vi "Unloading.vi"(8 "error In":errorcluster) -> (0 "error out":errorcluster)   [LabVIEW 2017]
uses:
  Controls/UNLOADING_DISPLAY.ctl
  Controls/Unload_Cyc_Data.ctl
  <vilib>/Utility/error.llb/DialogType.ctl
  Controls/QUEUE_STATES.ctl
  Controls/Unload_St.ctl
  <vilib>/Utility/file.llb/Read Delimited Spreadsheet (string).vi
  <vilib>/Instr/_visa.llb/VISA Configure Serial Port (Instr).vi
panel:
  out "EXPECTED SCAN CODE":string
  out "SCANNED CODE STATUS":bool
  out "DOOR OPEN":bool
  out "Cluster":T1
  out "CURRENT PLAN":T2
  out "all rows":string[][](array[string])
  out "logical AND":bool
  out "element":u16
  in  "Close _Door":bool
  out "raw scan code":string
  in  "BYPASS SCN":bool
  in  "String":string
  out "Scanner Comm":bool
  out "Stop scanner":bool
  out "CYCLE STATUS":string
  out "SCAN CODE:":string
  out "Selected Plan structure":string[][](table)
  out "Plan Selected:":string
  out "USER:-":string
  in  "Stop":bool
  out "DATE/TIME":string
  out "Screen Name":string
  # "DOOR NUMBER"
  # "SCANNED CODE"
  # "UNLOAD STATUS"
  # "DOOR NUMBER"
  # "SCANNED CODE"
  # "UNLOAD STATUS"
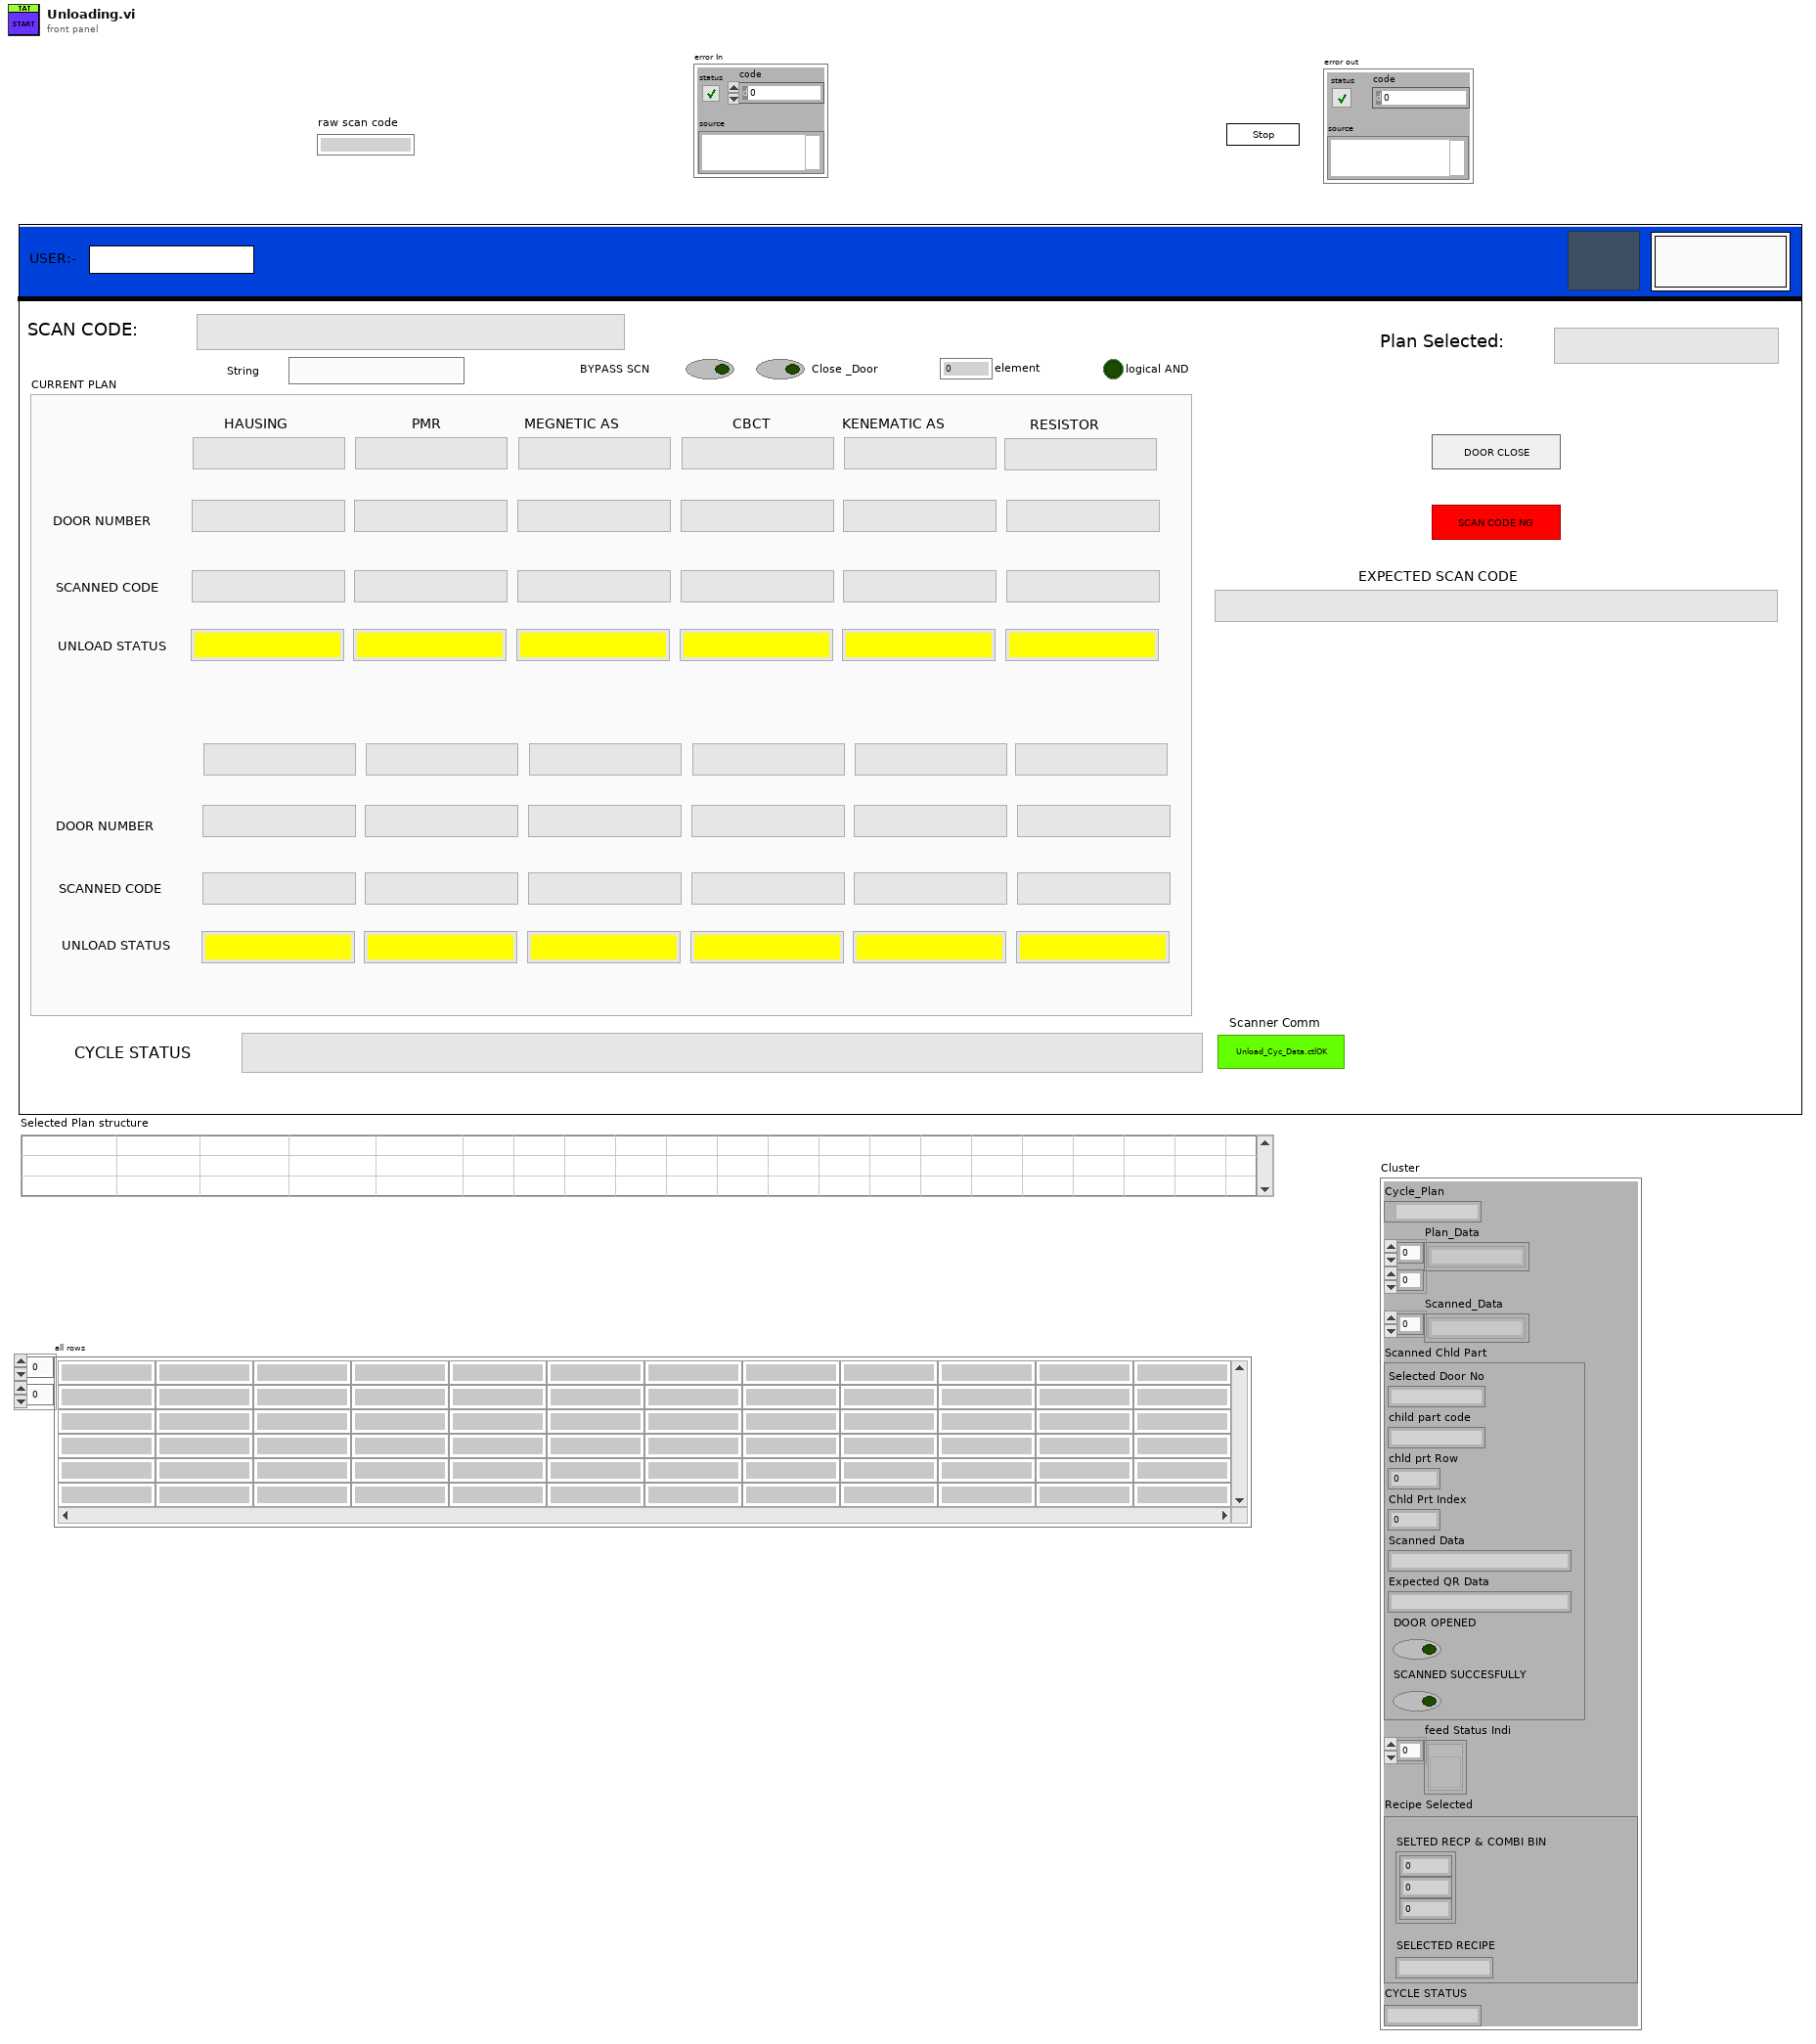
[diagram p1: front panel]
types:
  T1 = typedef "Unload_Cyc_Data.ctl" = cluster{"Cycle_Plan":path, "Plan_Data":string[][], "Scanned_Data":string[], "Scanned Chld Part":cluster{"Selected Door No":string, "child part code":string, "chld prt Row":i32, "Chld Prt Index":i32, "Scanned Data":string, "Expected QR Data":string, "DOOR OPENED":bool, "SCANNED SUCCESFULLY":bool}, "feed Status Indi":refnum<vi>[], "Recipe Selected":cluster{"SELTED RECP & COMBI BIN":cluster{"RECIPE INDEX":i32, "COMBI BIN":i32, "Section row no.":i32}, "SELECTED RECIPE":string}, "CYCLE STATUS":string}
  T2 = typedef "UNLOADING_DISPLAY.ctl" = cluster{"HAUSING":string, "PMR":string, "MEGNETIC AS":string, "CBCT":string, "KENEMATIC AS":string, "RESISTOR":string, "HAUSING DOOR":string, "PMR DOOR":string, "MAGNETIC AS DOOR":string, "CBCT DOOR":string, "KINEMATIC AS DOOR":string, "RESISTOR DOOR":string, "HAUSING SCAN QR":string, "PMR SCAN QR":string, "MAGNETIC SCAN QR":string, "CBCT SCAN QR":string, "KINEMATIC SCAN QR":string, "RESISTOR SCAN QR":string, "HAUSING UNLOAD STATUS":string, "PMR UNLOAD STATUS":string, "MAGNETIC AS UNLOAD STATUS":string, "CBCT UNLOAD STATUS":string, "KINEMATIC AS UNLOAD STATUS":string, "RESISTOR 1 UNLOAD STATUS":string, "HAUSING 2":string, "PMR 2":string, "MEGNETIC AS 2":string, "CBCT 2":string, "KENEMATIC AS 2":string, "RESISTOR 2":string, "HAUSING DOOR 4":string, "PMR DOOR 4":string, "MAGNETIC AS DOOR 4":string, "CBCT DOOR 4":string, "KINEMATIC AS DOOR 4":string, "RESISTOR 1 DOOR 4":string, "HAUSING 2 SCAN QR":string, "PMR 2 SCAN QR":string, "MAGNETIC 2 SCAN QR":string, "CBCT 2 SCAN QR":string, "KINEMATIC 2 SCAN QR":string, "RESISTOR 2 SCAN QR":string, "HAUSING UNLOAD STATUS 2":string, "PMR UNLOAD STATUS 2":string, "MAGNETIC AS UNLOAD STATUS 2":string, "CBCT UNLOAD STATUS 2":string, "KINEMATIC AS UNLOAD STATUS 2":string, "RESISTOR 1 UNLOAD STATUS 2":string}
  T3 = typedef "DialogType.ctl" = u16
  T4 = enum32{"invalid app kind", "Development System", "Run Time System", "Student Edition", "Embedded LabVIEW", "Evaluation", "Custom"}
  T5 = typedef "QUEUE_STATES.ctl" = enum16{"CREATE Q", "EN Q", "DE Q", "CLOSE Q"}
  T6 = cluster{"Printer IP":string, "PLC IP Address":string, "Scanner Com":refnum<visa-resource-name>}
  T7 = typedef "Unload_St.ctl" = enum16{"Int", "Int 2", "Wait", "Cluster_update", "Empty_Bin_Check", "Check_Section_to_Run", "Open_Door", "QR_Scanned", "Close_Door", "Error_Handler", "Stop"}
  T8 = cluster{"RECIPE INDEX":i32, "COMBI BIN":i32, "Section row no.":i32}
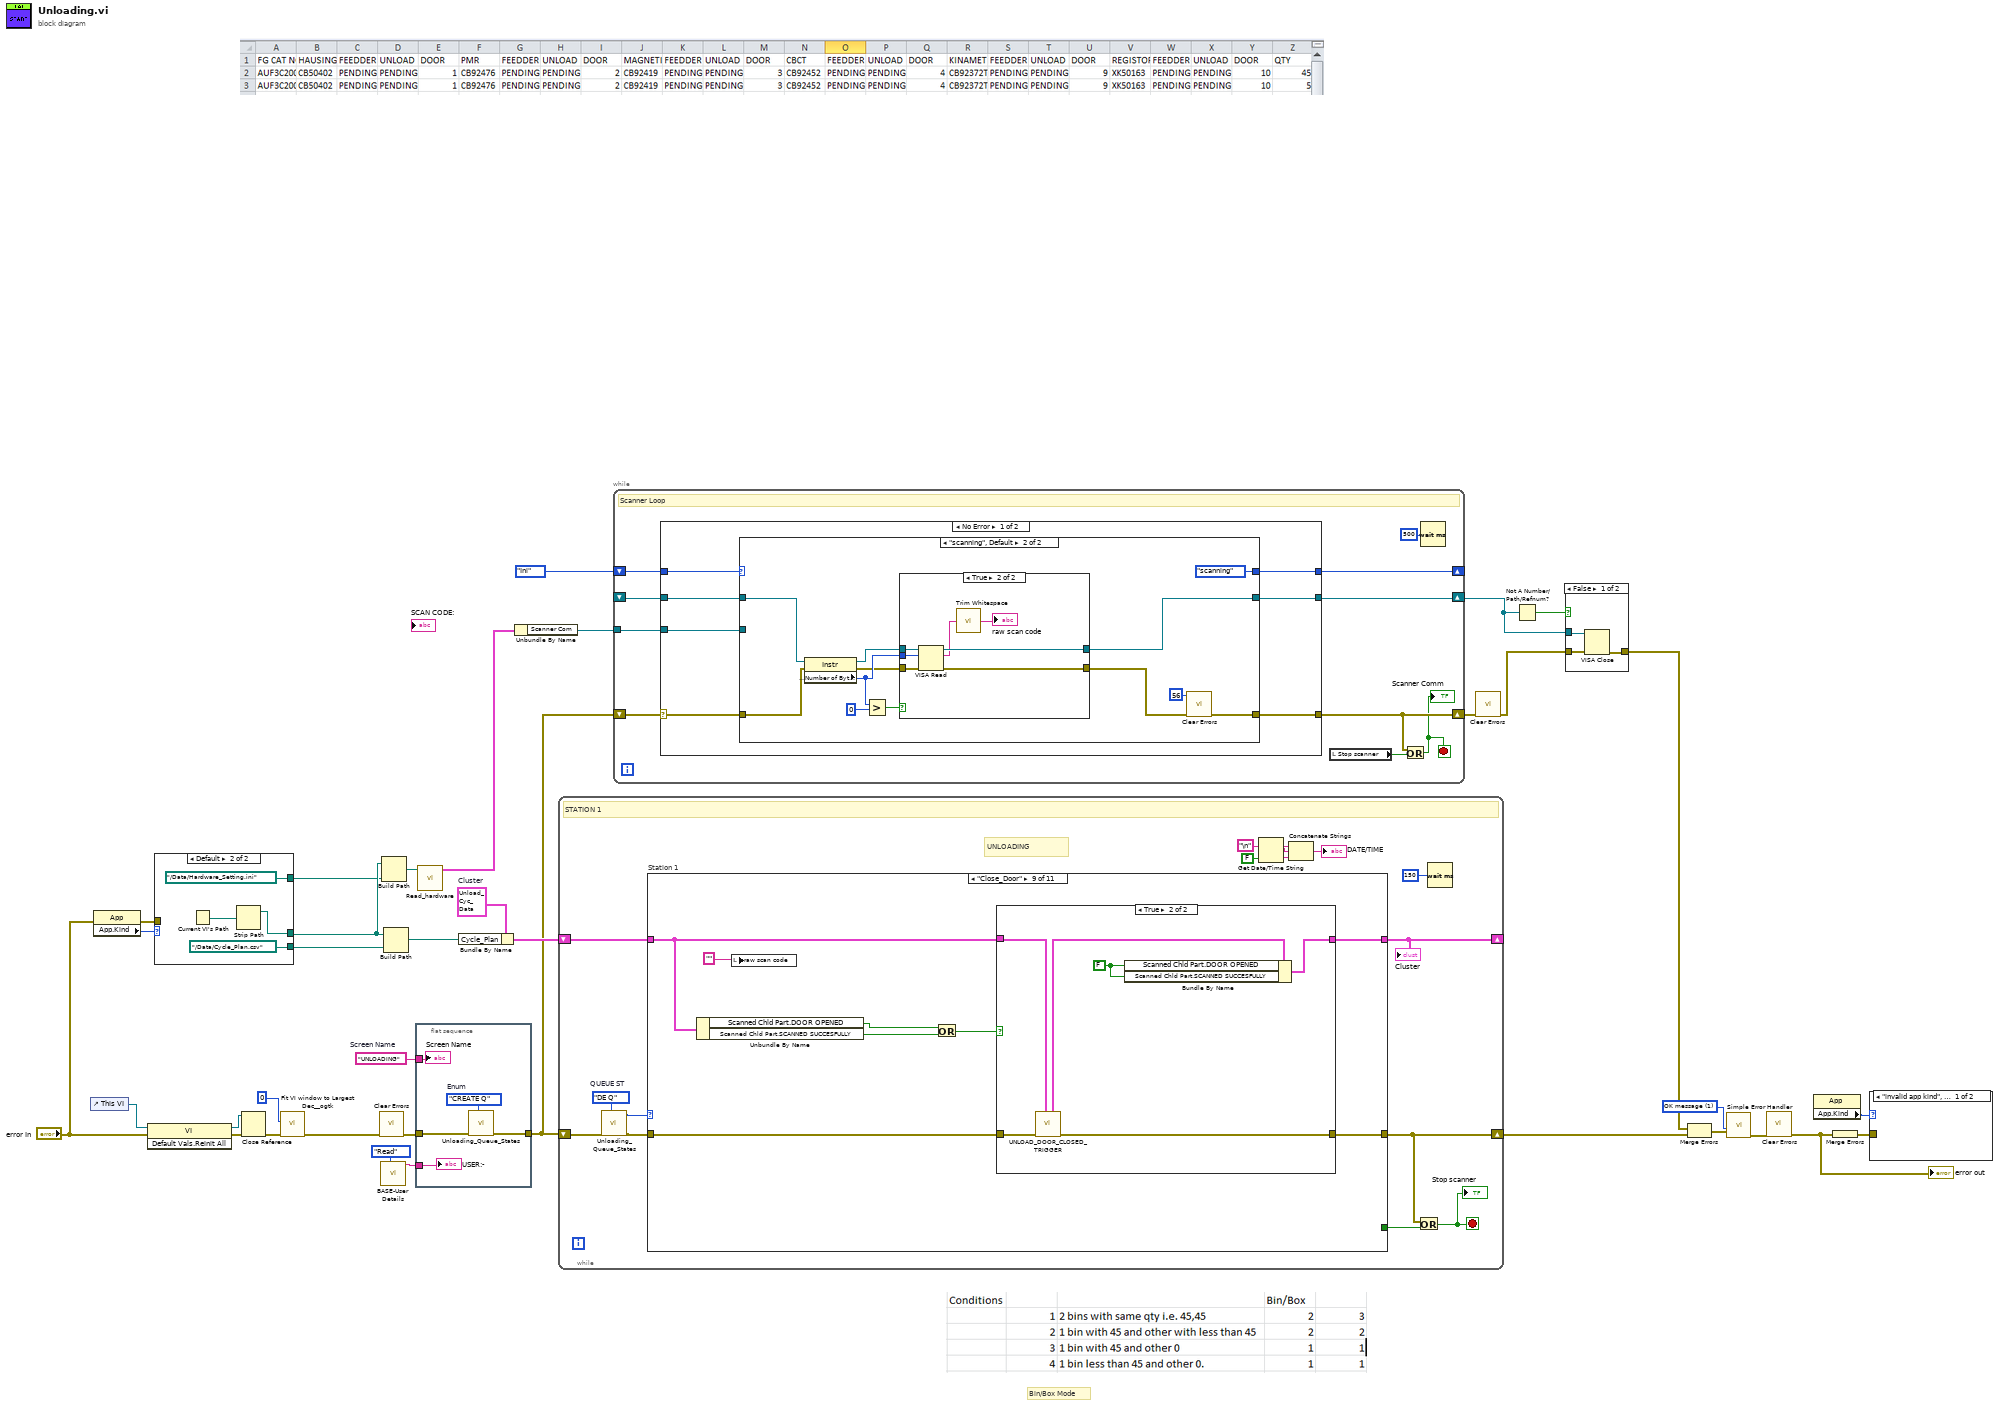
[diagram p0: block diagram]
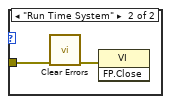
[diagram p2: hidden frame]
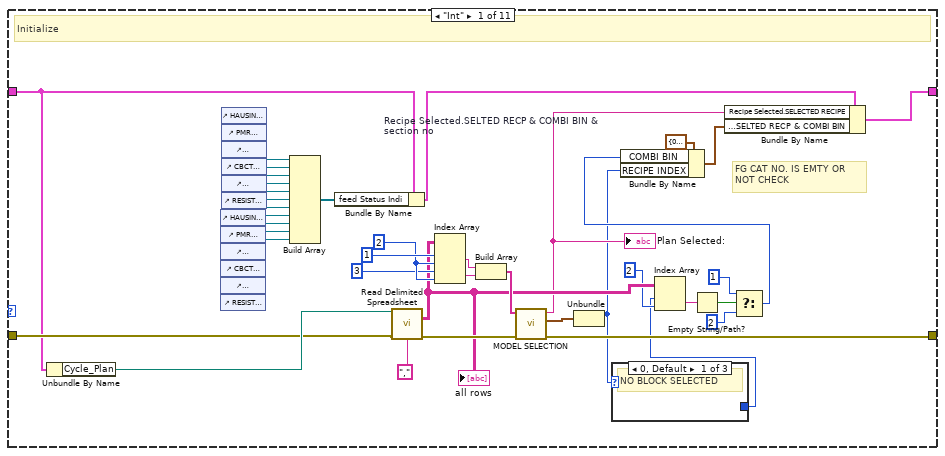
[diagram p3: hidden frame]
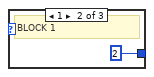
[diagram p4: hidden frame]
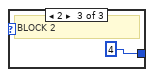
[diagram p5: hidden frame]
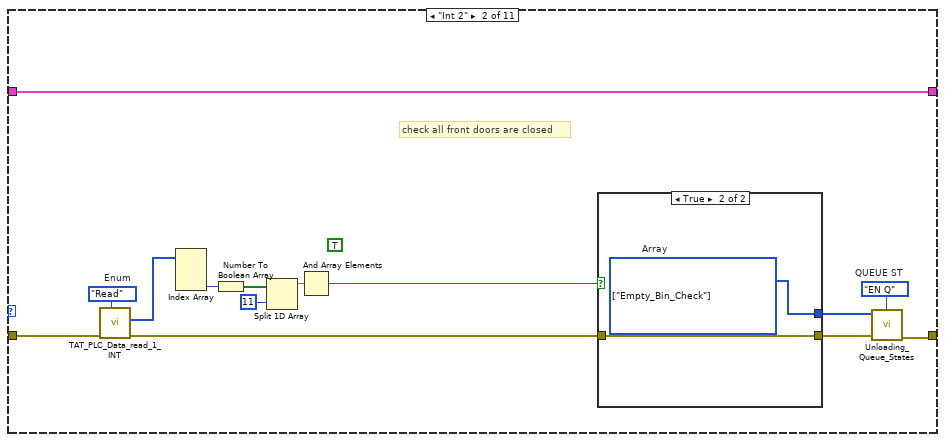
[diagram p6: hidden frame]
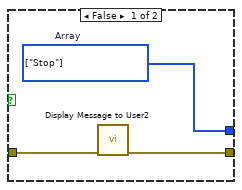
[diagram p7: hidden frame]
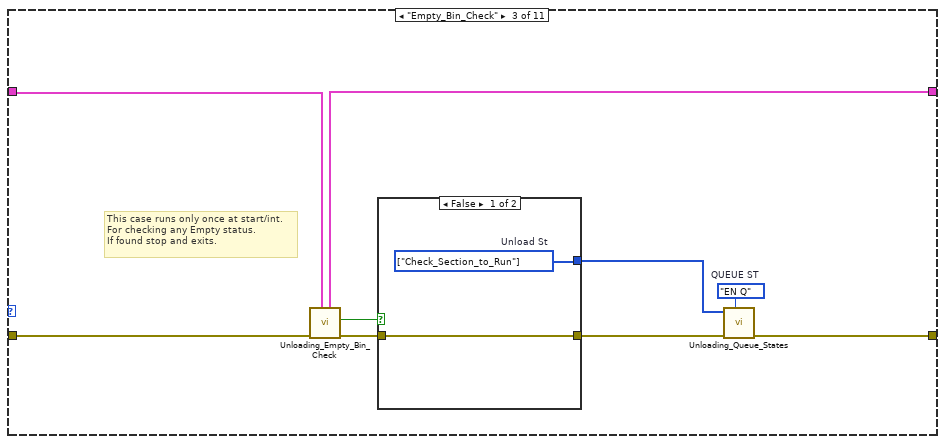
[diagram p8: hidden frame]
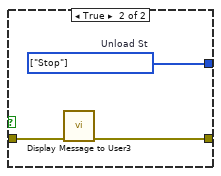
[diagram p9: hidden frame]
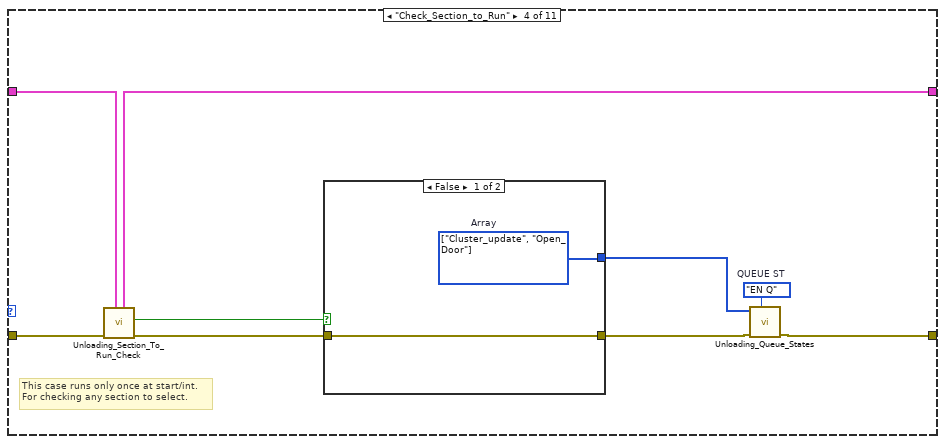
[diagram p10: hidden frame]
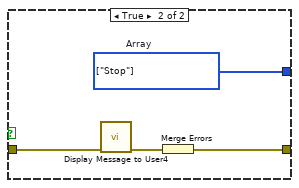
[diagram p11: hidden frame]
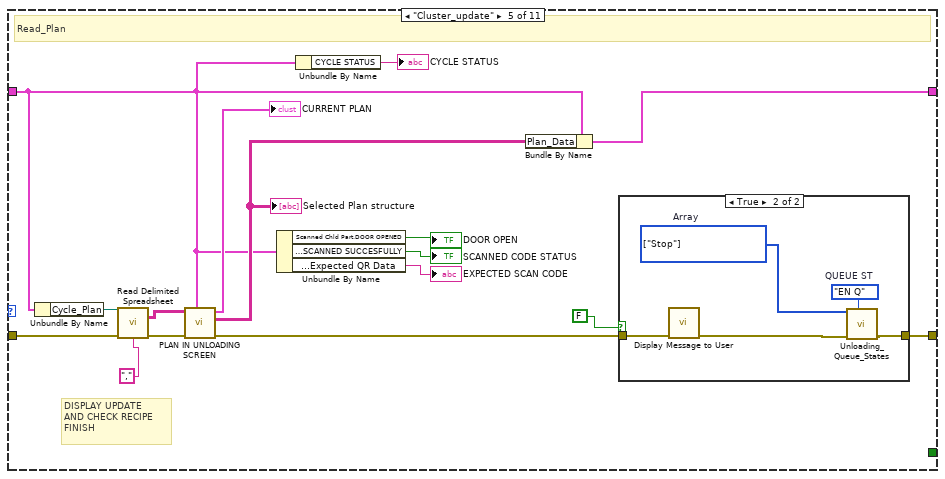
[diagram p12: hidden frame]
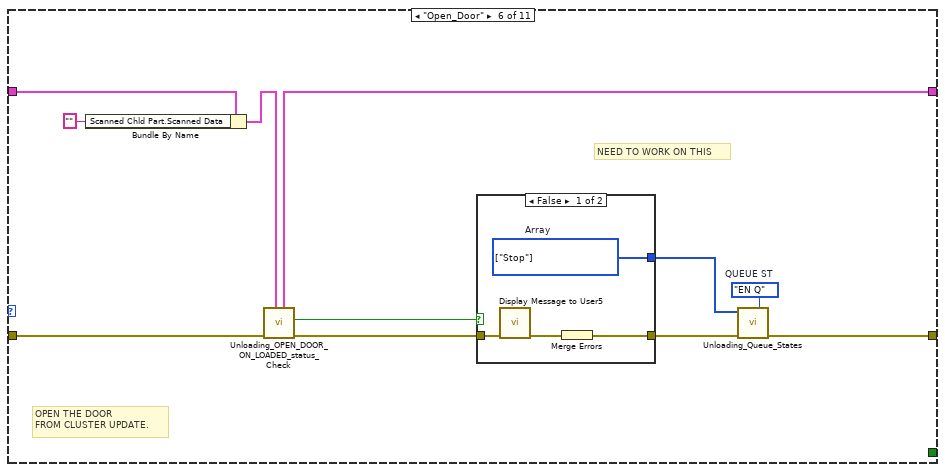
[diagram p14: hidden frame]
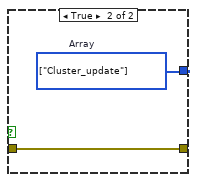
[diagram p15: hidden frame]
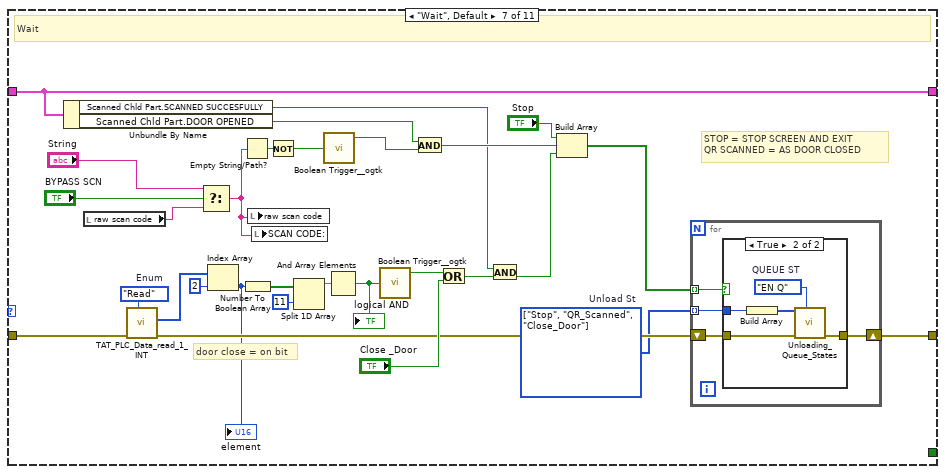
[diagram p16: hidden frame]
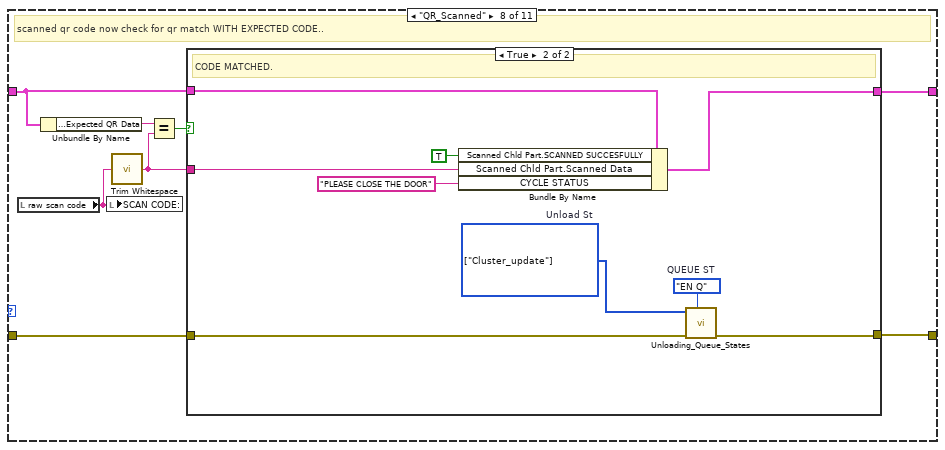
[diagram p18: hidden frame]
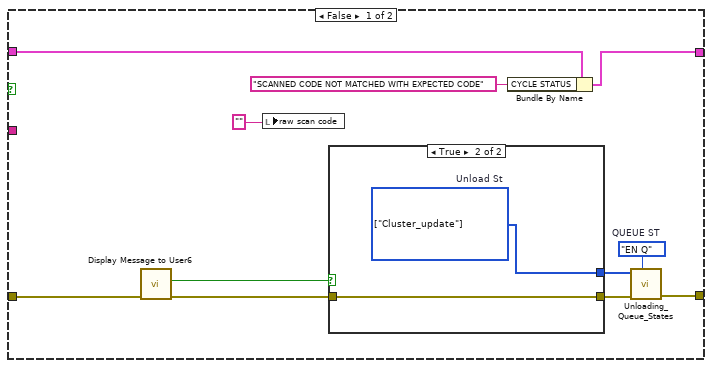
[diagram p19: hidden frame]
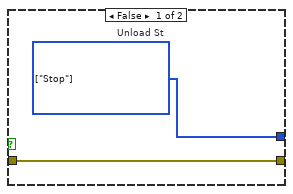
[diagram p20: hidden frame]
diagram:
  w1 = T1 {"Cycle_Plan"=path "", "Plan_Data"=[], "Scanned_Data"=[], "Scanned Chld Part"={"Selected Door No"="", "child part code"="", "chld prt Row"=0, "Chld Prt Index"=0, "Scanned Data"="", "Expected QR Data"="", "DOOR OPENED"=FALSE, "SCANNED SUCCESFULLY"=FALSE}, "feed Status Indi"=[], "Recipe Selected"={"SELTED RECP & COMBI BIN"={"RECIPE INDEX"=0, "COMBI BIN"=0, "Section row no."=0}, "SELECTED RECIPE"=""}, "CYCLE STATUS"=""}  # Cluster
  w18 = "UNLOADING"  # Screen Name
  w29 = T3 1 items=["no dialog", "OK message", "continue or stop message", "OK message + warnings", "continue/stop + warnings"] ("type of dialog (OK msg:1)")
  # "Bin/Box Mode"
  n1 = control-ref of="This VI"() -> (w36:refnum<vi>)
  n2 = property class="App"(error in="error In") -> (error out=w25:errorcluster, "App.Kind"=w27:T4)  [unwired: 1 in, 1 out]
  n3 = invoke class="VI" method="Default Vals.Reinit All"(reference=w36, error in="error In") -> (reference out=w34:refnum<vi>, error out=w35:errorcluster)  [unwired: 1 in, 1 out]
  n4 = case shown="Default" w27 {
    tunnel: [path "Data/Cycle_Plan.csv" ("path") path "../Data/Cycle_Plan.csv" ("path")] -> w26
    tunnel: [w37 w41] -> w7
    tunnel: w25 -> [_ _]
    tunnel: [path "Data/Hardware_Setting.ini" ("path") path "../Data/Hardware_Setting.ini" ("path")] -> w6
    frame "Run Time System" {
      n5 = call <vilib>:"Application Directory.vi"() -> ("Application Directory"=w37:path)
    }
    frame Default {
      n6 = Current VI's Path() -> (path=w42:path)
      n7 = Strip Path(path=w42) -> (stripped path=w41:path)  [unwired: 1 out]
    }
  }
  n8 = Close Reference(reference=w34, error in (no error)=w35) -> (error out=w33:errorcluster)
  n9 = call <userlib>:"Fit VI window to Largest Dec__ogtk.vi"("error in (no error)"=w33, "border spacing (2 px)"=0) -> ("error out"=w23:errorcluster)  [unwired: 4 in, 1 out]
  n10 = call <vilib>:"Clear Errors.vi"("error in (no error)"=w23) -> ("error out"=w11:errorcluster)  [unwired: 5 in, 1 out]
  n11 = call "BASE-User Details.vi"("Enum"=enum16{"Read", "Write"}."Read") -> ("User Name Out"=w30:string)  [unwired: 9 in, 1 out]
  n12 = Build Path(base path=w7, name or relative path=w6) -> (appended path=w5:path)
  n13 = Build Path(base path=w7, name or relative path=w26) -> (appended path=w20:path)
  n14 = flat-sequence {
    tunnel: [w45] -> w12
    tunnel: w11 -> [w46]
    tunnel: w30 -> [w48]
    tunnel: w18 -> [w47]
    frame #0 {
      w44 = QUEUE_STATES."CREATE Q"  # Enum
      n15 = call "Unloading_Queue_States.vi"("QUEUE ST"=w44, "error in"=w46) -> ("error OUT"=w45:errorcluster)  [unwired: 8 in, 1 out]
      "USER:-" <- w48
      "Screen Name" <- w47
    }
  }
  n16 = call "Read_hardware.vi"("configuration file path"=w5) -> ("data"=w9:T6)  [unwired: 10 in]
  n17 = Bundle By Name(cluster=w1, "Cycle_Plan"=w20) -> (w19:T1)
  n18 = Unbundle By Name(w9) -> ("Scanner Com"=w8:refnum<visa-resource-name>)
  n19 = while {
    shift-right: [w55] -> _
    shift-left: w19 -> [w56]
    shift-right: [w53] -> w10
    shift-left: w12 -> [w52]
    stop <- w54 stop-if-true
    w49 = QUEUE_STATES."DE Q"  # QUEUE ST
    # "UNLOADING"
    # "STATION 1"
    n20 = call "Unloading_Queue_States.vi"("QUEUE ST"=w49, "error in"=w52) -> ("error OUT"=w51:errorcluster, "Unload ST"=w50:T7)  [unwired: 8 in]
    n21 = case "Station 1" shown="\"Close_Door\"" w50 {
      tunnel: [_ _ _ _ _ _ _ _ _ _ TRUE] -> w57
      tunnel: [w80 w108 w128 w145 w158 w176 w218 w238 w269 w284 w288] -> w53
      tunnel: w51 -> [w98 w112 w132 w143 w167 w183 w209 w236 w270 w285 w289]
      tunnel: w56 -> [w89 w118 w131 w141 w156 w182 w196 w235 w268 w283 w290]
      tunnel: [w90 w118 w130 w140 w159 w181 w196 w237 w267 w283 w290] -> w55
      frame "Int" {
        w68 = T8 {"RECIPE INDEX"=0, "COMBI BIN"=0, "Section row no."=0}  # Recipe Selected.SELTED RECP & COMBI BIN & section no
        w95 = 2
        # "FG CAT NO. IS EMTY OR \nNOT CHECK"
        # "Initialize"
        n22 = Unbundle By Name(w89) -> ("Cycle_Plan"=w101:path)
        n23 = control-ref of="HAUSING UNLOAD STATUS 2"() -> (w73:refnum<vi>)
        n24 = control-ref of="PMR UNLOAD STATUS 2"() -> (w72:refnum<vi>)
        n25 = control-ref of="MAGNETIC AS UNLOAD STATUS 2"() -> (w71:refnum<vi>)
        n26 = control-ref of="CBCT UNLOAD STATUS 2"() -> (w70:refnum<vi>)
        n27 = control-ref of="KINEMATIC AS UNLOAD STATUS 2"() -> (w69:refnum<vi>)
        n28 = control-ref of="RESISTOR 1 UNLOAD STATUS 2"() -> ()  [unwired: 1 out]
        n29 = control-ref of="HAUSING UNLOAD STATUS"() -> (w79:refnum<vi>)
        n30 = control-ref of="PMR UNLOAD STATUS"() -> (w78:refnum<vi>)
        n31 = control-ref of="MAGNETIC AS UNLOAD STATUS"() -> (w77:refnum<vi>)
        n32 = control-ref of="CBCT UNLOAD STATUS"() -> (w76:refnum<vi>)
        n33 = control-ref of="KINEMATIC AS UNLOAD STATUS"() -> (w75:refnum<vi>)
        n34 = control-ref of="RESISTOR 1 UNLOAD STATUS"() -> (w74:refnum<vi>)
        n35 = Build Array(w79, w78, w77, w76, w75, w74, w73, w72, w71, w70, w69) -> (w102:refnum<vi>[])
        n36 = Bundle By Name(cluster=w89, "feed Status Indi"=w102) -> (w91:T1)
        n37 = call-poly <vilib>:"Read Delimited Spreadsheet.vi"("file path (dialog if empty)"=w101, "error in (no error)"=w98, "delimiter (\\t)"=",") -> ("all rows"=w88:string[][], "error out"=w97:errorcluster)  [unwired: 7 in, 4 out]
        "all rows" <- w88
        n38 = Index Array(array=w88, index (row) #1=1, index (col) #1=w95, index (row) #2=3, index (col) #2=w95) -> (element #1=w93:string, element #2=w92:string)
        n39 = Build Array(w93, w92) -> (w100:string[])
        n40 = call "MODEL SELECTION.vi"("error in (no error)"=w97, "Plan List"=w100) -> ("error out 2"=w80:errorcluster, "SELECTED RECIPE\nand COMBI OF BIN- INDEX"=w82:cluster{"RECIPE INDEX":i32, "COMBI BIN":i32}, "Plan Selected"=w81:string)  [unwired: 7 in]
        "Plan Selected:" <- w81
        n41 = Unbundle(w82) -> ("RECIPE INDEX"=w64:i32)  [unwired: 1 out]
        n42 = case shown="0, Default" w64 {
          tunnel: [_ 2 4] -> w65
          frame 0, Default {
            # "NO BLOCK SELECTED"
          }
          frame 1 {
            # "BLOCK 1"
          }
          frame 2 {
            # "BLOCK 2"
          }
        }
        n43 = Index Array(array=w88, index (row)=w65, index (col)=2) -> (element=w86:string)
        n44 = Empty String/Path?(string/path=w86) -> (empty?=w85:bool)
        n45 = Select(t=1, s=w85, f=2) -> (s? t:f=w66:i32)
        n46 = Bundle By Name(cluster=w68, "COMBI BIN"=w66, "RECIPE INDEX"=w64) -> (w67:T8)
        n47 = Bundle By Name(cluster=w91, "Recipe Selected.SELECTED RECIPE"=w81, "Recipe Selected.SELTED RECP & COMBI BIN"=w67) -> (w90:T1)
      }
      frame "Int 2" {
        (unwired) TRUE
        w110 = QUEUE_STATES."EN Q"  # QUEUE ST
        w117 = enum16{"Read", "Write"}."Read"  # Enum
        # "check all front doors are closed"
        n48 = call "TAT_PLC_Data_read_1_INT.vi"("Enum"=w117, "error in (no error)"=w112) -> ("error out"=w111:errorcluster, "Array 2"=w116:u16[])  [unwired: 8 in]
        n49 = Index Array(array=w116) -> (element #3=w105:u16)  [unwired: 3 in, 2 out]
        n50 = Number To Boolean Array(number=w105) -> (Boolean array=w115:bool[])
        n51 = Split 1D Array(array=w115, index=11) -> (first subarray=w113:bool[])  [unwired: 1 out]
        n52 = And Array Elements(Boolean array=w113) -> (logical AND=w106:bool)
        n53 = case shown="True" w106 {
          tunnel: w111 -> [w121 w123]
          tunnel: [w120 w123] -> w107
          tunnel: [w119 w122] -> w109
          frame False {
            w119 = T7[] [enum."Stop"] items=["Int", "Int 2", "Wait", "Cluster_update", "Empty_Bin_Check", "Check_Section_to_Run", "Open_Door", "QR_Scanned", "Close_Door", "Error_Handler", "Stop"]  # Array
            n54 = call "Display Message to User2"("error in (no error)"=w121) -> ("error out"=w120:errorcluster)  [unwired: 9 in, 1 out]
          }
          frame True {
            w122 = T7[] [enum."Empty_Bin_Check"] items=["Int", "Int 2", "Wait", "Cluster_update", "Empty_Bin_Check", "Check_Section_to_Run", "Open_Door", "QR_Scanned", "Close_Door", "Error_Handler", "Stop"]  # Array
          }
        }
        n55 = call "Unloading_Queue_States.vi"("QUEUE ST"=w110, "error in"=w107, "Unload St"=w109) -> ("error OUT"=w108:errorcluster)  [unwired: 7 in, 1 out]
      }
      frame "Empty_Bin_Check" {
        w127 = QUEUE_STATES."EN Q"  # QUEUE ST
        # "This case runs only once at start/int.\nFor checking any Empty status.\nIf found stop and exits."
        n56 = call "Unloading_Empty_Bin_Check.vi"("Cluster DATA IN"=w131, "error in (no error)"=w132) -> ("error out"=w129:errorcluster, "EMPTY FOUND ?"=w124:bool, "Cluster DATA OUT"=w130:T1)  [unwired: 7 in]
        n57 = case shown="False" w124 {
          tunnel: w129 -> [w134 w137]
          tunnel: [w133 w136] -> w126
          tunnel: [w134 w135] -> w125
          frame False {
            w133 = T7[] [enum."Check_Section_to_Run"] items=["Int", "Int 2", "Wait", "Cluster_update", "Empty_Bin_Check", "Check_Section_to_Run", "Open_Door", "QR_Scanned", "Close_Door", "Error_Handler", "Stop"]  # Unload St
          }
          frame True {
            w136 = T7[] [enum."Stop"] items=["Int", "Int 2", "Wait", "Cluster_update", "Empty_Bin_Check", "Check_Section_to_Run", "Open_Door", "QR_Scanned", "Close_Door", "Error_Handler", "Stop"]  # Unload St
            n58 = call "Display Message to User3"("error in (no error)"=w137) -> ("error out"=w135:errorcluster)  [unwired: 9 in, 1 out]
          }
        }
        n59 = call "Unloading_Queue_States.vi"("QUEUE ST"=w127, "error in"=w125, "Unload St"=w126) -> ("error OUT"=w128:errorcluster)  [unwired: 7 in, 1 out]
      }
      frame "Check_Section_to_Run" {
        w146 = QUEUE_STATES."EN Q"  # QUEUE ST
        # "This case runs only once at start/int.\nFor checking any section to select."
        n60 = call "Unloading_Section_To_Run_Check.vi"("Cluster DATA IN"=w141, "error in (no error)"=w143) -> ("error out"=w142:errorcluster, "FULLY UNLOADED FOUND ?"=w138:bool, "Cluster DATA OUT"=w140:T1)  [unwired: 7 in]
        n61 = case shown="False" w138 {
          tunnel: [w148 w152] -> w144
          tunnel: w142 -> [w147 w150]
          tunnel: [w147 w151] -> w139
          frame False {
            w148 = T7[] [enum."Cluster_update", enum."Open_Door"] items=["Int", "Int 2", "Wait", "Cluster_update", "Empty_Bin_Check", "Check_Section_to_Run", "Open_Door", "QR_Scanned", "Close_Door", "Error_Handler", "Stop"]  # Array
          }
          frame True {
            w152 = T7[] [enum."Stop"] items=["Int", "Int 2", "Wait", "Cluster_update", "Empty_Bin_Check", "Check_Section_to_Run", "Open_Door", "QR_Scanned", "Close_Door", "Error_Handler", "Stop"]  # Array
            n62 = call "Display Message to User4"("error in (no error)"=w150) -> ("error out"=w149:errorcluster)  [unwired: 9 in, 1 out]
            n63 = Merge Errors(w149) -> (w151:errorcluster)
          }
        }
        n64 = call "Unloading_Queue_States.vi"("QUEUE ST"=w146, "error in"=w139, "Unload St"=w144) -> ("error OUT"=w145:errorcluster)  [unwired: 7 in, 1 out]
      }
      frame "Cluster_update" {
        # "DISPLAY UPDATE\nAND CHECK RECIPE\nFINISH"
        # "Read_Plan"
        n65 = Unbundle By Name(w156) -> ("Cycle_Plan"=w166:path)
        n66 = call-poly <vilib>:"Read Delimited Spreadsheet.vi"("file path (dialog if empty)"=w166, "error in (no error)"=w167, "delimiter (\\t)"=",") -> ("all rows"=w162:string[][], "error out"=w164:errorcluster)  [unwired: 7 in, 4 out]
        n67 = call "PLAN IN UNLOADING SCREEN.vi"("LOOP DATA IN"=w156, "error IN"=w164, "PLAN In"=w162) -> ("error out"=w163:errorcluster, "PLAN Out"=w160:string[][], "CURRENT PLAN"=→"CURRENT PLAN":T2)  [unwired: 4 in, 1 out]
        "Selected Plan structure" <- w160
        n68 = Unbundle By Name(w156) -> ("Scanned Chld Part.DOOR OPENED"=→"DOOR OPEN":bool, "Scanned Chld Part.SCANNED SUCCESFULLY"=→"SCANNED CODE STATUS":bool, "Scanned Chld Part.Expected QR Data"=→"EXPECTED SCAN CODE":string)
        n69 = Unbundle By Name(w156) -> ("CYCLE STATUS"=→"CYCLE STATUS":string)
        n70 = Bundle By Name(cluster=w156, "Plan_Data"=w160) -> (w159:T1)
        n71 = case shown="True" FALSE {
          tunnel: w163 -> [w169 w174]
          tunnel: [w169 w171] -> w158
          frame False {
          }
          frame True {
            w170 = T7[] [enum."Stop"] items=["Int", "Int 2", "Wait", "Cluster_update", "Empty_Bin_Check", "Check_Section_to_Run", "Open_Door", "QR_Scanned", "Close_Door", "Error_Handler", "Stop"]  # Array
            w173 = QUEUE_STATES."EN Q"  # QUEUE ST
            n72 = call "Display Message to User"("error in (no error)"=w174) -> ("error out"=w172:errorcluster)  [unwired: 9 in, 1 out]
            n73 = call "Unloading_Queue_States.vi"("QUEUE ST"=w173, "error in"=w172, "Unload St"=w170) -> ("error OUT"=w171:errorcluster)  [unwired: 7 in, 1 out]
          }
        }
      }
      frame "Open_Door" {
        w178 = QUEUE_STATES."EN Q"  # QUEUE ST
        # "NEED TO WORK ON THIS"
        # "OPEN THE DOOR\nFROM CLUSTER UPDATE."
        n74 = Bundle By Name(cluster=w182, "Scanned Chld Part.Scanned Data"="") -> (w185:T1)
        n75 = call "Unloading_OPEN_DOOR_ON_LOADED_status_Check.vi"("CYCLE DATA IN"=w185, "error in"=w183) -> ("error out"=w177:errorcluster, "search valid ?"=w175:bool, "CYCLE DATA OUT"=w181:T1)  [unwired: 7 in]
        n76 = case shown="False" w175 {
          tunnel: [w189 w191] -> w180
          tunnel: w177 -> [w187 w190]
          tunnel: [w188 w190] -> w179
          frame False {
            w189 = T7[] [enum."Stop"] items=["Int", "Int 2", "Wait", "Cluster_update", "Empty_Bin_Check", "Check_Section_to_Run", "Open_Door", "QR_Scanned", "Close_Door", "Error_Handler", "Stop"]  # Array
            n77 = call "Display Message to User5"("error in (no error)"=w187) -> ("error out"=w186:errorcluster)  [unwired: 9 in, 1 out]
            n78 = Merge Errors(w186) -> (w188:errorcluster)
          }
          frame True {
            w191 = T7[] [enum."Cluster_update"] items=["Int", "Int 2", "Wait", "Cluster_update", "Empty_Bin_Check", "Check_Section_to_Run", "Open_Door", "QR_Scanned", "Close_Door", "Error_Handler", "Stop"]  # Array
          }
        }
        n79 = call "Unloading_Queue_States.vi"("QUEUE ST"=w178, "error in"=w179, "Unload St"=w180) -> ("error OUT"=w176:errorcluster)  [unwired: 7 in, 1 out]
      }
      frame "Wait", Default {
        w192 = T7[] [enum."Stop", enum."QR_Scanned", enum."Close_Door"] items=["Int", "Int 2", "Wait", "Cluster_update", "Empty_Bin_Check", "Check_Section_to_Run", "Open_Door", "QR_Scanned", "Close_Door", "Error_Handler", "Stop"]  # Unload St
        w207 = enum16{"Read", "Write"}."Read"  # Enum
        # "STOP = STOP SCREEN AND EXIT\nQR SCANNED = AS DOOR CLOSED"
        # "door close = on bit"
        # "Wait"
        n80 = Unbundle By Name(w196) -> ("Scanned Chld Part.SCANNED SUCCESFULLY"=w193:bool, "Scanned Chld Part.DOOR OPENED"=w195:bool)
        n81 = local read "raw scan code"() -> (w214:string)
        n82 = call "TAT_PLC_Data_read_1_INT.vi"("Enum"=w207, "error in (no error)"=w209) -> ("error out"=w208:errorcluster, "Array 2"=w206:u16[])  [unwired: 8 in]
        n83 = Select(t="String", s="BYPASS SCN", f=w214) -> (s? t:f=w211:string)
        n84 = Index Array(array=w206, index=2) -> (element=w203:u16)
        "element" <- w203
        n85 = Empty String/Path?(string/path=w211) -> (empty?=w217:bool)
        n86 = Number To Boolean Array(number=w203) -> (Boolean array=w202:bool[])
        n87 = local write "raw scan code"(w211) -> ()
        n88 = local write "SCAN CODE:"(w211) -> ()
        n89 = Not(x=w217) -> (.not. x?=w210:bool)
        n90 = Split 1D Array(array=w202, index=11) -> (first subarray=w200:bool[])  [unwired: 1 out]
        n91 = call <userlib>:"Boolean Trigger__ogtk.vi"("Boolean Input"=w210) -> ("Rising Edge"=w205:bool)  [unwired: 1 in, 1 out]
        n92 = And Array Elements(Boolean array=w200) -> (logical AND=w197:bool)
        "logical AND" <- w197
        n93 = call <userlib>:"Boolean Trigger__ogtk.vi"("Boolean Input"=w197) -> ("Rising Edge"=w204:bool)  [unwired: 1 in, 1 out]
        n94 = And(x=w195, y=w205) -> (x .and. y?=w198:bool)
        n95 = Or(x=w204, y="Close _Door") -> (x .or. y?=w212:bool)
        n96 = And(x=w193, y=w212) -> (x .and. y?=w194:bool)
        n97 = Build Array("Stop", w198, w194) -> (w215:bool[])
        n98 = for {
          shift-right: [w223] -> w218
          shift-left: w208 -> [w224]
          tunnel: w215 -> [w222] mode=indexing
          tunnel: w192 -> [w221] mode=indexing
          n99 = case shown="True" w222 {
            tunnel: w224 -> [w225 w228]
            tunnel: [w225 w229] -> w223
            tunnel: w221 -> [_ w230]
            frame False {
            }
            frame True {
              w227 = QUEUE_STATES."EN Q"  # QUEUE ST
              n100 = Build Array(w230) -> (w226:T7[])
              n101 = call "Unloading_Queue_States.vi"("QUEUE ST"=w227, "error in"=w228, "Unload St"=w226) -> ("error OUT"=w229:errorcluster)  [unwired: 7 in, 1 out]
            }
          }
        }
      }
      frame "QR_Scanned" {
        # "scanned qr code now check for qr match WITH EXPECTED CODE.."
        n102 = local read "raw scan code"() -> (w233:string)
        n103 = Unbundle By Name(w235) -> ("Scanned Chld Part.Expected QR Data"=w234:string)
        n104 = local write "SCAN CODE:"(w233) -> ()
        n105 = call <vilib>:"Trim Whitespace.vi"("string"=w233) -> ("trimmed string"=w231:string)  [unwired: 1 in]
        n106 = Equal?(x=w234, y=w231) -> (x = y?=w232:bool)
        n107 = case shown="True" w232 {
          tunnel: [w241 w255] -> w238
          tunnel: [w248 w261] -> w237
          tunnel: w236 -> [w246 w256]
          tunnel: w235 -> [w249 w262]
          tunnel: w231 -> [_ w259]
          frame False {
            w242 = QUEUE_STATES."EN Q"  # QUEUE ST
            n108 = call "Display Message to User6"("error in (no error)"=w246) -> ("error out"=w245:errorcluster, "RETRY"=w244:bool)  [unwired: 9 in]
            n109 = local write "raw scan code"("") -> ()
            n110 = case shown="True" w244 {
              tunnel: w245 -> [w251 w253]
              tunnel: [w251 w253] -> w240
              tunnel: [w250 w252] -> w239
              frame False {
                w250 = T7[] [enum."Stop"] items=["Int", "Int 2", "Wait", "Cluster_update", "Empty_Bin_Check", "Check_Section_to_Run", "Open_Door", "QR_Scanned", "Close_Door", "Error_Handler", "Stop"]  # Unload St
              }
              frame True {
                w252 = T7[] [enum."Cluster_update"] items=["Int", "Int 2", "Wait", "Cluster_update", "Empty_Bin_Check", "Check_Section_to_Run", "Open_Door", "QR_Scanned", "Close_Door", "Error_Handler", "Stop"]  # Unload St
              }
            }
            n111 = Bundle By Name(cluster=w249, "CYCLE STATUS"="SCANNED CODE NOT MATCHED WITH EXPECTED CODE") -> (w248:T1)
            n112 = call "Unloading_Queue_States.vi"("QUEUE ST"=w242, "error in"=w240, "Unload St"=w239) -> ("error OUT"=w241:errorcluster)  [unwired: 7 in, 1 out]
          }
          frame True {
            w257 = QUEUE_STATES."EN Q"  # QUEUE ST
            w254 = T7[] [enum."Cluster_update"] items=["Int", "Int 2", "Wait", "Cluster_update", "Empty_Bin_Check", "Check_Section_to_Run", "Open_Door", "QR_Scanned", "Close_Door", "Error_Handler", "Stop"]  # Unload St
            # "CODE MATCHED."
            n113 = Bundle By Name(cluster=w262, "Scanned Chld Part.SCANNED SUCCESFULLY"=TRUE, "Scanned Chld Part.Scanned Data"=w259, "CYCLE STATUS"="PLEASE CLOSE THE DOOR") -> (w261:T1)
            n114 = call "Unloading_Queue_States.vi"("QUEUE ST"=w257, "error in"=w256, "Unload St"=w254) -> ("error OUT"=w255:errorcluster)  [unwired: 7 in, 1 out]
          }
        }
      }
      frame "Close_Door" {
        n115 = Unbundle By Name(w268) -> ("Scanned Chld Part.DOOR OPENED"=w264:bool, "Scanned Chld Part.SCANNED SUCCESFULLY"=w266:bool)
        n116 = local write "raw scan code"("") -> ()
        n117 = Or(x=w264, y=w266) -> (x .or. y?=w265:bool)
        n118 = case shown="True" w265 {
          tunnel: w270 -> [w276 w282]
          tunnel: [w271 w281] -> w269
          tunnel: w268 -> [w275 w280]
          tunnel: [w275 w278] -> w267
          frame False {
            w273 = T7[] [enum."Stop"] items=["Int", "Int 2", "Wait", "Cluster_update", "Empty_Bin_Check", "Check_Section_to_Run", "Open_Door", "QR_Scanned", "Close_Door", "Error_Handler", "Stop"]  # Array
            w274 = QUEUE_STATES."EN Q"  # QUEUE ST
            n119 = call "Display Message to User7"("error in (no error)"=w276) -> ("error out"=w272:errorcluster)  [unwired: 9 in, 1 out]
            n120 = call "Unloading_Queue_States.vi"("QUEUE ST"=w274, "error in"=w272, "Unload St"=w273) -> ("error OUT"=w271:errorcluster)  [unwired: 7 in, 1 out]
          }
          frame True {
            w277 = FALSE
            n121 = call "UNLOAD_DOOR_CLOSED_TRIGGER.vi"("CYCLE DATA IN"=w280, "error in (no error)"=w282) -> ("error out"=w281:errorcluster, "CYCLE DATA OUT"=w279:T1)  [unwired: 8 in]
            n122 = Bundle By Name(cluster=w279, "Scanned Chld Part.DOOR OPENED"=w277, "Scanned Chld Part.SCANNED SUCCESFULLY"=w277) -> (w278:T1)
          }
        }
      }
      frame "Error_Handler" {
        n123 = call "STATION_1_STATUS.vi"("error in (no error)"=w285, "STATUS"="CYCLE STARTED" ("Cycle Status")) -> ("error out"=w284:errorcluster)  [unwired: 9 in]
      }
      frame "Stop" {
        w287 = QUEUE_STATES."CLOSE Q"  # QUEUE ST
        n124 = call "Unloading_Queue_States.vi"("QUEUE ST"=w287, "error in"=w289) -> ("error OUT"=w288:errorcluster)  [unwired: 8 in, 1 out]
      }
    }
    "Cluster" <- w55
    n125 = Get Date/Time String(want seconds? (F)=FALSE) -> (date string=w61:string, time string=w60:string)  [unwired: 2 in]
    n126 = Concatenate Strings(w61, "\n", w60) -> (→"DATE/TIME":string)
    n127 = Or(x=w53, y=w57) -> (x .or. y?=w54:bool)
    "Stop scanner" <- w54
    n128 = Wait (ms)(milliseconds to wait=u32 150) -> ()  [unwired: 1 out]
  }
  n129 = while {
    shift-right: [w300] -> w16
    shift-left: w12 -> [w301]
    shift-right: [w298] -> _
    shift-left: enum16{"Ini", "scanning", "Close"}."Ini" -> [w299]
    tunnel: w8 -> [w297]
    shift-right: [w296] -> w13
    shift-left: _ -> [w295]
    stop <- w294 stop-if-true
    # "Scanner Loop"
    n130 = case shown="No Error" w301 {
      selector: w301 -> [w308 w338]
      tunnel: [w307 w337] -> w300
      tunnel: w299 -> [w306 _]
      tunnel: [w305 enum16{"Ini", "scanning", "Close"}."scanning"] -> w298
      tunnel: w297 -> [w304 _]
      tunnel: [w303 w335] -> w296
      tunnel: w295 -> [w302 w335]
      frame No Error {
        n131 = case shown="\"scanning\", Default" w306 {
          tunnel: w308 -> [w312 w316]
          tunnel: [w311 w324] -> w307
          tunnel: [enum16{"Ini", "scanning", "Close"}."scanning" enum16{"Ini", "scanning", "Close"}."scanning"] -> w305
          tunnel: w304 -> [w310 _]
          tunnel: [w309 w314] -> w303
          tunnel: w302 -> [_ w317]
          frame "Ini" {
            n132 = call-poly "VISA Configure Serial Port"("VISA resource name"=w310, "error in (no error)"=w312) -> ("VISA resource name out"=w309:refnum<visa-resource-name>, "error out"=w311:errorcluster)  [unwired: 12 in]
          }
          frame "scanning", Default {
            n133 = property class="Instr"(reference=w317, error in=w316) -> (reference out=w319:refnum<visa-resource-name>, error out=w320:errorcluster, "Serial Settings:Number of Bytes at Serial Port"=w321:u32)
            n134 = Greater?(x=w321, y=u32 0) -> (0:w322:bool)
            n135 = case shown="True" w322 {
              tunnel: w319 -> [w327 w334]
              tunnel: w320 -> [w326 w333]
              tunnel: w321 -> [_ w332]
              tunnel: [w327 w331] -> w314
              tunnel: [w326 w329] -> w315
              frame False {
              }
              frame True {
                n136 = VISA Read(VISA resource name=w334, byte count=w332, error in (no error)=w333) -> (VISA resource name out=w331:refnum<visa-resource-name>, read buffer=w330:string, error out=w329:errorcluster)  [unwired: 1 out]
                n137 = call <vilib>:"Trim Whitespace.vi"("string"=w330) -> ("trimmed string"=→"raw scan code":string)  [unwired: 1 in]
              }
            }
            n138 = call <vilib>:"Clear Errors.vi"("error in (no error)"=w315, "specific error code to clear (0: all)"=56) -> ("error out"=w324:errorcluster)  [unwired: 4 in, 1 out]
          }
        }
      }
      frame Error {
        n139 = Unbundle By Name(w338) -> ("code"=w339:i32)
        n140 = case shown="1" w339 {
          tunnel: w338 -> [w343 w345]
          tunnel: [w341 w344] -> w337
          frame 0, Default {
            w340 = T3 2 items=["no dialog", "OK message", "continue or stop message", "OK message + warnings", "continue/stop + warnings"] ("type of dialog (OK msg:1)")
            n141 = call <vilib>:"Simple Error Handler.vi"("type of dialog (OK msg:1)"=w340, "error in (no error)"=w343) -> ("error out"=w342:errorcluster)  [unwired: 3 in, 4 out]
            n142 = call <vilib>:"Clear Errors.vi"("error in (no error)"=w342) -> ("error out"=w341:errorcluster)  [unwired: 5 in, 1 out]
          }
          frame 1 {
            w346 = "THIS ERROR OCCURED AS SCREEN 1 IS NOT CONNECTED OR OFF"  # source
            # "Monitor not present/Off/disconnected"
            n143 = Bundle By Name(cluster=w345, "source"=w346) -> (w344:errorcluster)
          }
        }
      }
    }
    n144 = local read "Stop scanner"() -> (w292:bool)
    n145 = Or(x=w300, y=w292) -> (x .or. y?=w294:bool)
    "Scanner Comm" <- w294
    n146 = Wait (ms)(milliseconds to wait=u32 500) -> ()  [unwired: 1 out]
  }
  n147 = call <vilib>:"Clear Errors.vi"("error in (no error)"=w16) -> ("error out"=w14:errorcluster)  [unwired: 5 in, 1 out]
  n148 = Not A Number/Path/Refnum?(number/path/refnum=w13) -> (NaN/Path/Refnum?=w15:bool)
  n149 = case shown="False" w15 {
    tunnel: w14 -> [w349 w350]
    tunnel: w13 -> [w347 _]
    tunnel: [w348 w350] -> w4
    frame False {
      n150 = VISA Close(VISA resource name=w347, error in (no error)=w349) -> (error out=w348:errorcluster)
    }
    frame True {
    }
  }
  n151 = Merge Errors(w4, w10) -> (w32:errorcluster)
  n152 = call <vilib>:"Simple Error Handler.vi"("type of dialog (OK msg:1)"=w29, "error in (no error)"=w32) -> ("error out"=w3:errorcluster)  [unwired: 3 in, 4 out]
  n153 = call <vilib>:"Clear Errors.vi"("error in (no error)"=w3) -> ("error out"=w2:errorcluster)  [unwired: 5 in, 1 out]
  "error out" <- w2
  n154 = property class="App"() -> ("App.Kind"=w28:T4)  [unwired: 2 in, 2 out]
  n155 = Merge Errors(w2) -> (w21:errorcluster)
  n156 = case shown="\"invalid app kind\", Default" w28 {
    tunnel: w21 -> [_ w352]
    frame "invalid app kind", Default {
    }
    frame "Run Time System" {
      n157 = call <vilib>:"Clear Errors.vi"("error in (no error)"=w352) -> ("error out"=w351:errorcluster)  [unwired: 5 in, 1 out]
      n158 = invoke class="VI" method="FP.Close"(error in=w351) -> ()  [unwired: 2 in, 3 out]
    }
  }
